vi "Mod_OFDM_Close_Configuration_Files.vi"(11 "error in (no error)":errorcluster) -> (15 "error out":errorcluster)   [LabVIEW 2010]
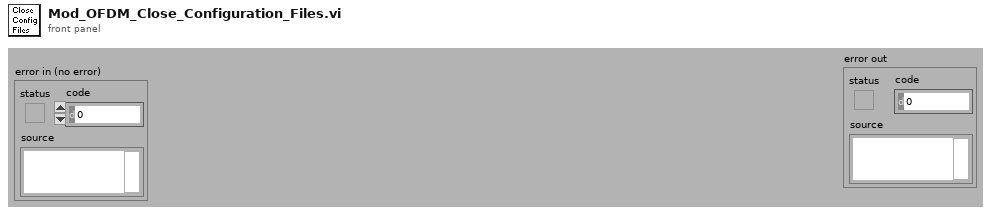
[diagram p1: front panel]
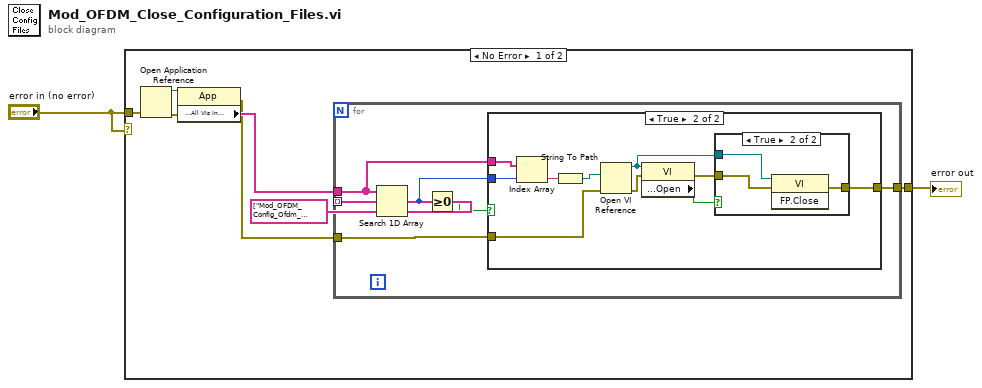
[diagram p0: block diagram]
diagram:
  n1 = case shown="No Error" "error in (no error)" {
    tunnel: [w6 w31] -> w2
    tunnel: "error in (no error)" -> [w5 w31]
    frame No Error {
      n2 = Open Application Reference(8:w5) -> (0:w4:errorcluster, 3:w9:refnum<vi>)  [unwired: 3 in]
      n3 = property class="App"(reference=w9, error in=w4) -> (error out=w3:errorcluster, "Application:All VIs In Memory"=w7:string[])  [unwired: 1 out]
      n4 = for {
        tunnel: string[] ["Mod_OFDM_Config_Ofdm_Parameters.vi", "Mod_OFDM_Config_Data_Source.vi", "Mod_OFDM_Config_Modulator_Source.vi", "Mod_OFDM_Config_Ofdm_Symbol.vi", "Mod_OFDM_Config_Ofdm_Frame.vi", "Mod_OFDM_Config_Pulse_Shaping.vi", "Mod_OFDM_Config_Waveform_generation.vi", ""] -> [w12] mode=indexing
        tunnel: w7 -> [w14]
        tunnel: w3 -> [w11]
        tunnel: [w10] -> w6
        n5 = Search 1D Array(1D array=w14, element=w12) -> (index of element=w13:i32)  [unwired: 1 in]
        n6 = Greater Or Equal To 0?(x=w13) -> (x >= 0?=w15:bool)
        n7 = case shown="True" w15 {
          tunnel: w14 -> [_ w26]
          tunnel: w13 -> [_ w25]
          tunnel: w11 -> [w16 w22]
          tunnel: [w16 w17] -> w10
          frame False {
          }
          frame True {
            n8 = Index Array(array=w26, index=w25) -> (element=w24:string)
            n9 = String To Path(string=w24) -> (path=w23:path)
            n10 = Open VI Reference(vi path=w23, error in (no error)=w22) -> (vi reference=w20:refnum<vi>, error out=w19:errorcluster)  [unwired: 4 in]
            n11 = property class="VI"(reference=w20, error in=w19) -> (error out=w18:errorcluster, "Front Panel Window:Open"=w21:bool)  [unwired: 1 out]
            n12 = case shown="True" w21 {
              tunnel: w20 -> [_ w30]
              tunnel: w18 -> [w27 w29]
              tunnel: [w27 w28] -> w17
              frame False {
              }
              frame True {
                n13 = invoke class="VI" method="FP.Close"(reference=w30, error in=w29) -> (error out=w28:errorcluster)  [unwired: 1 in, 2 out]
              }
            }
          }
        }
      }
    }
    frame Error {
    }
  }
  "error out" <- w2
